vi "GPI-Join Sequences.vi"() -> ()   [LabVIEW 2015]
doc: "Combines two Glimpse video sequences into a single sequence that has the frames in chronological order based on time stamps."
uses:
  Header2 file data.ctl
  GLIMPSE Globals.vi
panel:
  in  "Number of acquisition files":i32=10
  out "Input Sequences Progress (%)":dbl[](array[slide]) scale=0.0..100.0
  out "Output frame number":i32(slide) scale=0.0..68.0
  in  "Radio Buttons":enum32{"New button", "Over-write button"}(radio)
  in  "Save into new directory:":path=path "d:/1.glimpse"
  in  "Over-write exisitng:":path=path "d:/1.glimpse"
  in  "Sequences to Join":path[](array[path])
  in  "Exit":bool
  in  "Go!":bool
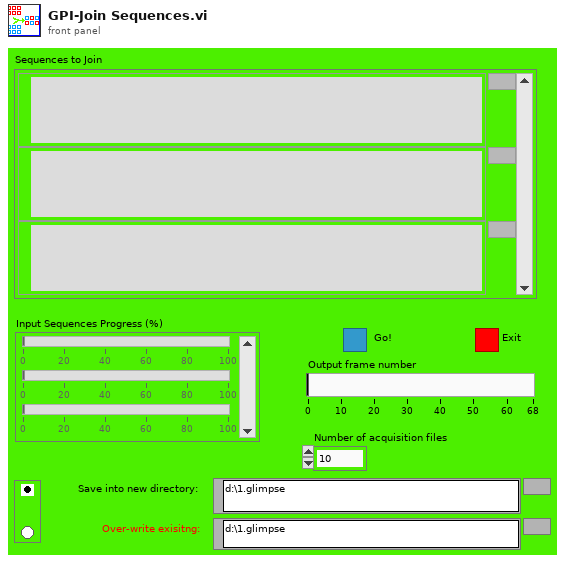
[diagram p1: front panel]
types:
  T1 = typedef "Header2 file data.ctl" = cluster{"Camera":string, "Microscope":string, "Microscope software version":string, "Laser names":string[], "Filter names":string[], "Lasers array":u16[][], "Filter array":u16[], "Flow rate array":dbl[], "Temperature array":dbl[], "Field array":u16[], "Is header2 info present?":bool, "Description Info":string, "Stage xyz array":dbl[][]}
  T2 = typedef "Header file data.ctl" = cluster{"Frames Acquired":u32, "Region width":i32, "Region height":i32, "Element 0 of TTB":u32, "time of 1st frame, \nsec since 1/1/04":dbl, "TTB Array (ms)":u32[], "Offsets Array":T3, "Pixel depth":u32}
  T3 = typedef "Offset table.ctl" = cluster{"offset":T4, "file number":T5}[]
  T4 = typedef "Offset.ctl" = i32
  T5 = typedef "file number.ctl" = u8
  T6 = typedef "IMAQ Image.ctl" = refnum<image>
  T7 = typedef "Sequence files handle.ctt" = cluster{"Sequence files directory path":path, "Sequence files refnum array":refnum<file>[]}
  T8 = typedef "Image Type" = u32
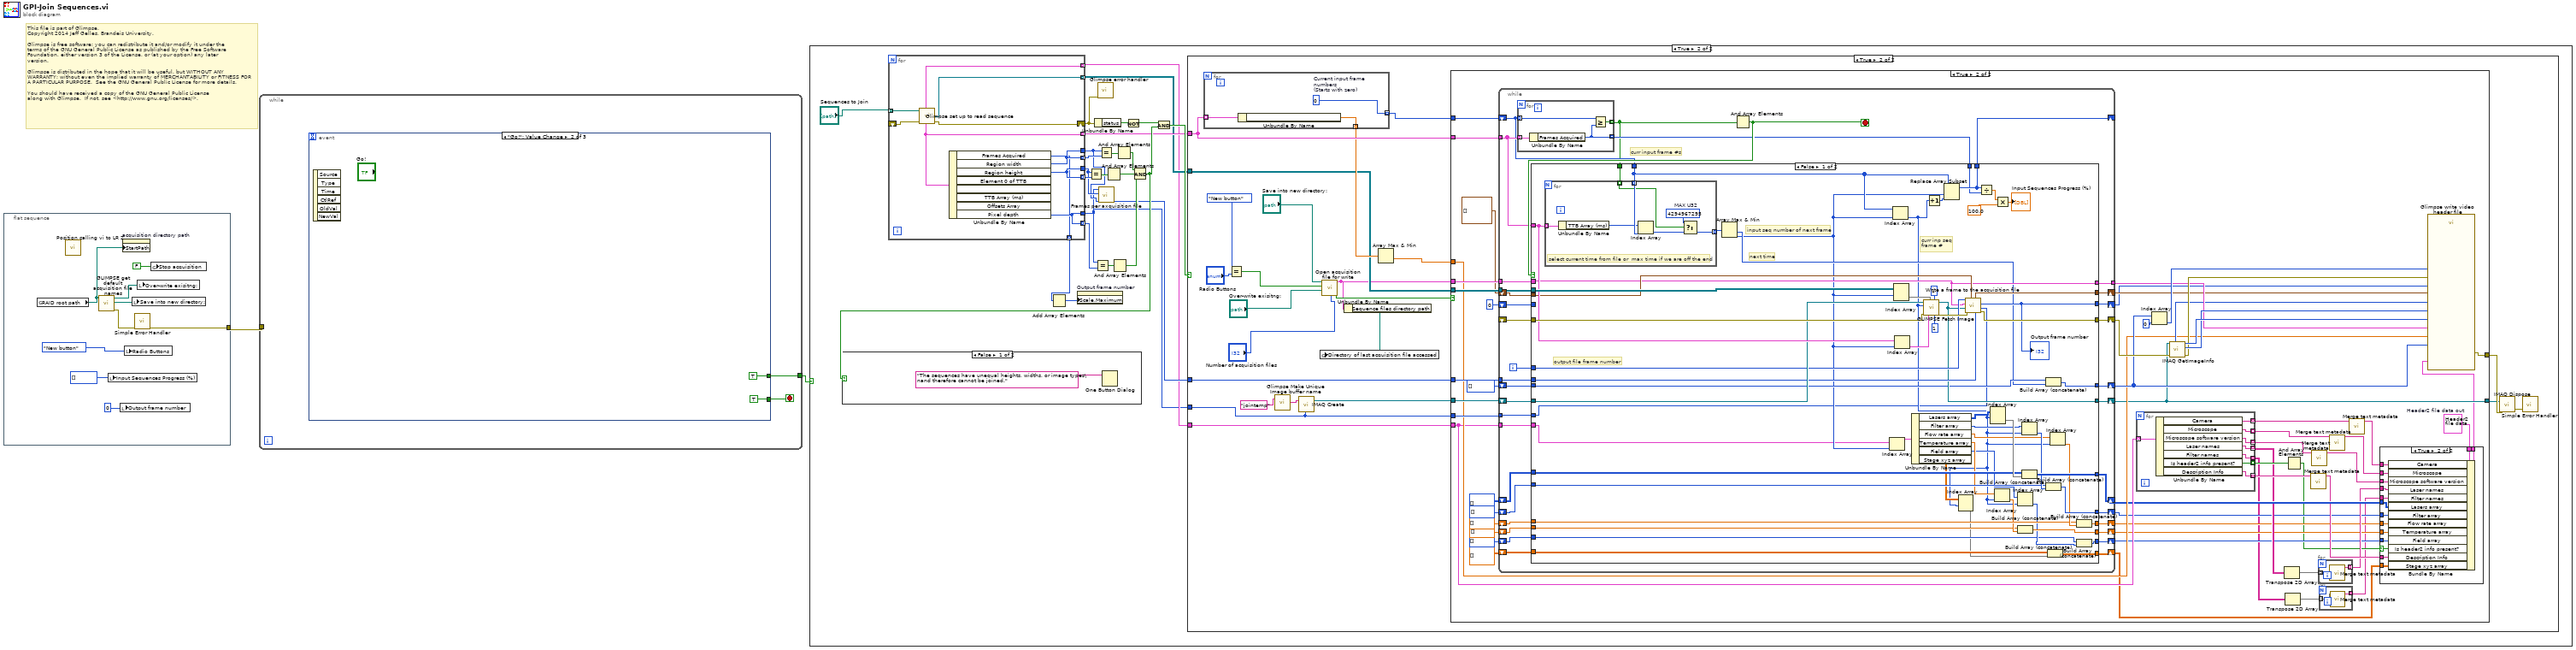
[diagram p0: block diagram]
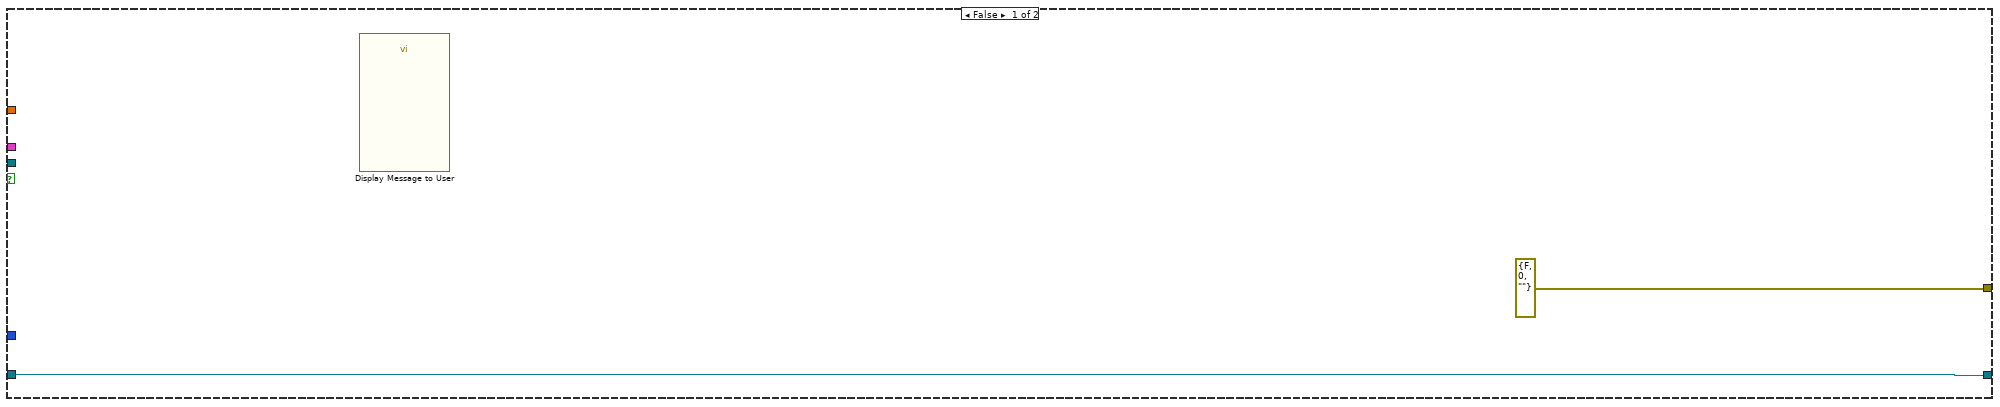
[diagram p4: hidden frame]
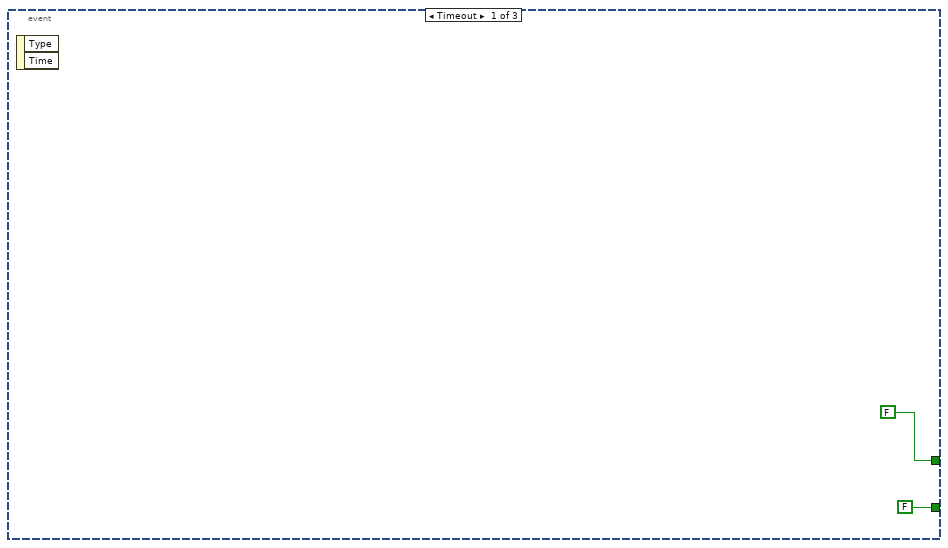
[diagram p8: hidden frame]
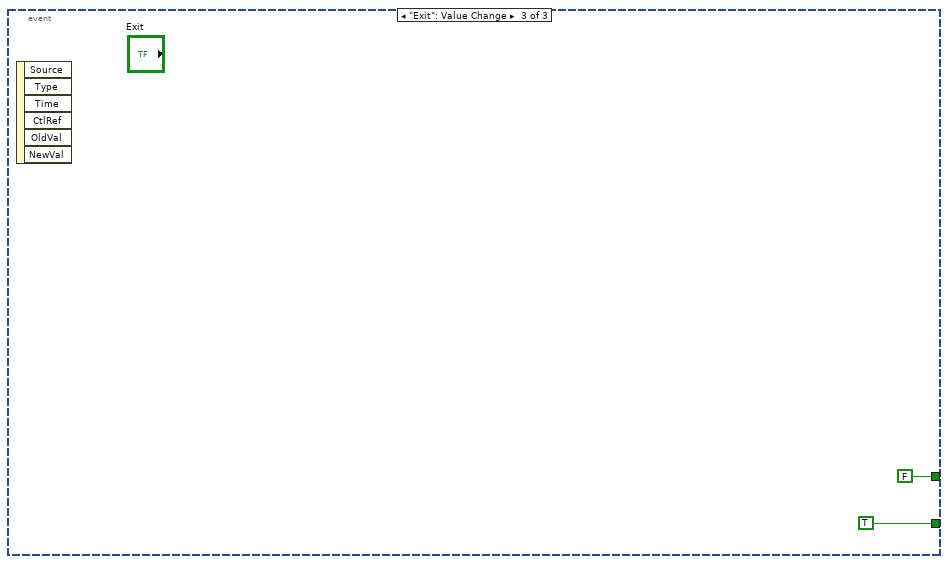
[diagram p9: hidden frame]
diagram:
  # "This file is part of Glimpse. \nCopyright 2014 Jeff Gelles, Brandeis University.    \n\nGlimpse is free software: you can redistribute it and/or modify it under the \nterms of the GNU General Public License as published by the Free Software \nFoundation, either version 3 of the License, or (at your option) any later \nversion.\n\nGlimpse is distributed in the hope that it will be useful, but WITHOUT ANY \nWARRANTY; without even the implied warranty of MERCHANTABILITY or FITNESS FOR \nA PARTICULAR PURPOSE.  See the GNU General Public License for more details.\n\nYou should have received a copy of the GNU General Public License\nalong with Glimpse.  If not, see <http://www.gnu.org/licenses/>."
  n1 = flat-sequence {
    tunnel: [w6] -> w1
    frame #0 {
      n2 = global read "GLIMPSE Globals.vi" "RAID root path"() -> (w3:path)
      n3 = call "Position calling vi to LR 2.vi"() -> ()  [unwired: 2 in, 4 out]
      n4 = call "GLIMPSE get default acquisition file names.vi"("RAID root path"=w3) -> ("error out"=w9:errorcluster, "next directory path"=w10:path, "last directory path"=w11:path)  [unwired: 1 in, 5 out]
      n5 = local write "Input Sequences Progress (%)"(u64[] [] ("Input Sequences Progress (%)")) -> ()
      n6 = local write "Output frame number"(0 ("Output frame number")) -> ()
      n7 = property on="acquisition directory path" class="Path"("StartPath"=w3) -> ()  [unwired: 2 in, 2 out]
      n8 = local write "Radio Buttons"(enum32{"New button", "Over-write button"}."New button" ("Radio Buttons")) -> ()
      n9 = local write "Save into new directory:"(w10) -> ()
      n10 = call <vilib>:"Simple Error Handler.vi"("error in (no error)"=w9) -> ("error out"=w6:errorcluster)  [unwired: 1 in, 7 out]
      n11 = local write "Over-write exisitng:"(w11) -> ()
      n12 = global write "GLIMPSE Globals.vi" "Stop acquisition"(FALSE ("Stop acquisition")) -> ()
    }
  }
  n13 = while {
    tunnel: [w12] -> w2
    tunnel: w1 -> [_]
    stop <- w13 stop-if-true
    n14 = event shown="[1] \"Go!\": Value Change" {
      selector: _ -> [_ _ _]
      dyn-events: _ -> [_ _ _]
      timeout: _ -> [_ _ _]
      tunnel: [FALSE TRUE TRUE] -> w13
      tunnel: [FALSE ("Boolean") TRUE FALSE] -> w12
      event Timeout {
        n15 = event-data() -> ()  [unwired: 3 out]
      }
      event "Go!": Value Change {
        n16 = event-data() -> ()  [unwired: 7 out]
      }
      event "Exit": Value Change {
        n17 = event-data() -> ()  [unwired: 7 out]
      }
    }
  }
  n18 = case shown="True" w2 {
    frame False {
    }
    frame True {
      n19 = for {
        tunnel: "Sequences to Join" -> [w282] mode=indexing
        shift-right: [w280] -> w33
        shift-left: _ -> [w281]
        tunnel: [w279] -> w29 mode=indexing
        tunnel: [w278] -> w26
        tunnel: [w277] -> w27
        tunnel: [w276] -> w37 mode=indexing
        tunnel: [w278] -> w42 mode=indexing
        tunnel: [w277] -> w39 mode=indexing
        tunnel: [w276] -> w20
        tunnel: [w275] -> w28 mode=indexing
        tunnel: [w274] -> w23 mode=indexing
        tunnel: [w273] -> w21 mode=indexing
        n20 = call "Glimpse set up to read sequence.vi"("acquisition directory path"=w282, "error in"=w281) -> ("Header2 file data out"=w273:T1, "Header file data out"=w279:T2, "Acquisition refnum array"=w275:refnum<file>[], "error out"=w280:errorcluster)  [unwired: 2 out]
        n21 = Unbundle By Name(w279) -> ("Frames Acquired"=w274:u32, "Region width"=w278:i32, "Region height"=w277:i32, "Pixel depth"=w276:u32)  [unwired: 4 out]
      }
      n22 = Add Array Elements(numeric array=w23) -> (sum=w24:u32)
      n23 = property on="Output frame number" class="Slide (strict)"("Scale.Maximum"=w24) -> ()  [unwired: 2 in, 2 out]
      n24 = Equal?(x=w27, y=w39) -> (x = y?=w40:bool[])
      n25 = Unbundle By Name(w33) -> ("status"=w32:bool)
      n26 = Equal?(x=w20, y=w37) -> (x = y?=w38:bool[])
      n27 = call "Glimpse error handler.vi"("error in"=w33) -> ()  [unwired: 1 in, 6 out]
      n28 = call "Frames per axquisition file.vi"("Output frame width"=w26, "Output frame height"=w27, "Pixel depth"=w20) -> ("Frames per acquisition file"=w25:i32)  [unwired: 3 in, 1 out]
      n29 = Equal?(x=w26, y=w42) -> (x = y?=w41:bool[])
      n30 = And Array Elements(Boolean array=w40) -> (logical AND=w35:bool)
      n31 = And Array Elements(Boolean array=w38) -> (logical AND=w36:bool)
      n32 = And Array Elements(Boolean array=w41) -> (logical AND=w34:bool)
      n33 = Not(x=w32) -> (.not. x?=w22:bool)
      n34 = Compound Arithmetic op=AND(w34, w35, w36) -> (w31:bool)
      n35 = case shown="False" w31 {
        frame False {
          n36 = One Button Dialog(message="The sequences have unequal heights, widths, or image types\nand therefore cannot be joined.") -> ()  [unwired: 2 out]
        }
        frame True {
        }
      }
      n37 = And(x=w22, y=w31) -> (x .and. y?=w30:bool)
      n38 = case shown="True" w30 {
        tunnel: w29 -> [_ w59]
        tunnel: w28 -> [_ w57]
        tunnel: w20 -> [_ w53]
        tunnel: w25 -> [_ w52]
        tunnel: w21 -> [_ w45]
        frame False {
        }
        frame True {
          n39 = for {
            tunnel: [w271] -> w66 mode=indexing
            tunnel: w59 -> [w270] mode=indexing
            tunnel: [w269] -> w58 mode=indexing
            w271 = u64 0  # Current input frame  numbers (Starts with zero)
            n40 = Unbundle By Name(w270) -> ("time of 1st frame, \nsec since 1/1/04"=w269:dbl)
          }
          n41 = Equal?(x=enum32{"New button", "Over-write button"}."New button", y="Radio Buttons") -> (x = y?=w61:bool)
          n42 = call "Glimpse Make Unique Image buffer name.vi"("Buffer  base name"="jointemp" ("Image Name")) -> ("Image Name"=w56:string)  [unwired: 1 out]
          n43 = call "IMAQ Create"("Image Name"=w56, "Image Type"=w53) -> ("New Image"=w54:T6)  [unwired: 2 in, 2 out]
          n44 = call "Open acquisition file for write.vi"("Number of acquisition files"="Number of acquisition files", "Existing directory to over-write"="Over-write exisitng:", "Use new?"=w61, "New directory to create"="Save into new directory:") -> ("OK?"=w60:bool, "Sequence files handle"=w47:T7)  [unwired: 5 out]
          n45 = Unbundle By Name(w47) -> ("Sequence files directory path"=w46:path)
          n46 = global write "GLIMPSE Globals.vi" "Directory of last acquisition file accessed"(w46) -> ()
          n47 = Array Max & Min(array=w58) -> (min value=w51:dbl)  [unwired: 3 out]
          n48 = case shown="True" w60 {
            tunnel: w66 -> [_ w123]
            tunnel: w59 -> [_ w122]
            tunnel: w57 -> [_ w121]
            tunnel: w54 -> [w68 w120]
            tunnel: w47 -> [_ w119]
            tunnel: w53 -> [_ w118]
            tunnel: w52 -> [_ w116]
            tunnel: w51 -> [_ w103]
            tunnel: [errorcluster {"status"=FALSE, "code"=0, "source"=""} ("error out") w102] -> w50
            tunnel: [w68 w101] -> w49
            tunnel: w45 -> [_ w99]
            frame False {
              n49 = call "Display Message to User"() -> ()  [unwired: 3 in, 9 out]
            }
            frame True {
              w97 = T1 {"Camera"="", "Microscope"="", "Microscope software version"="", "Laser names"=[], "Filter names"=[], "Lasers array"=[], "Filter array"=[], "Flow rate array"=[], "Temperature array"=[], "Field array"=[], "Is header2 info present?"=FALSE, "Description Info"="", "Stage xyz array"=[]}  # Header2 file data out
              n50 = while {
                tunnel: w122 -> [w185]
                shift-right: [w173] -> _
                shift-left: w123 -> [w184]
                tunnel: w121 -> [w183]
                shift-right: [w181] -> w111
                shift-left: _ -> [w182]
                shift-right: [w172] -> w101
                shift-left: w120 -> [w180]
                tunnel: w119 -> [w179]
                tunnel: w118 -> [w177]
                shift-right: [w176] -> w104
                shift-left: cluster{"offset":i32, "file number":u8}[] [] ("Offset table out") -> [w175]
                tunnel: w116 -> [w174]
                shift-right: [w171] -> w107
                shift-left: u32[] [] -> [w170]
                shift-right: [w169] -> w100
                shift-left: u32 0 ("Last frame number written out") -> [w168]
                tunnel: [w167] -> w106
                tunnel: w99 -> [w165]
                shift-right: [w164] -> w90
                shift-left: u16[][] [] -> [w163]
                shift-right: [w162] -> w83
                shift-left: u16[] [] -> [w161]
                shift-right: [w160] -> w82
                shift-left: dbl[] [] -> [w159]
                shift-right: [w158] -> w81
                shift-left: dbl[] [] -> [w157]
                shift-right: [w156] -> w80
                shift-left: u16[] [] -> [w155]
                shift-right: [w153] -> w75
                shift-left: dbl[][] [] -> [w154]
                i -> [w178]
                stop <- w186 stop-if-true
                # "curr input frame #s"
                n51 = for {
                  tunnel: w184 -> [w265] mode=indexing
                  tunnel: w185 -> [w268] mode=indexing
                  tunnel: [w267] -> w152 mode=indexing
                  tunnel: [w266] -> w166 mode=indexing
                  n52 = Unbundle By Name(w268) -> ("Frames Acquired"=w266:u32)
                  n53 = Greater Or Equal?(x=w265, y=w266) -> (x >= y?=w267:bool)
                }
                n54 = And Array Elements(Boolean array=w152) -> (logical AND=w186:bool)
                n55 = case shown="False" w186 {
                  tunnel: w185 -> [w238 _]
                  tunnel: w184 -> [w229 w258]
                  tunnel: w183 -> [w243 _]
                  tunnel: w182 -> [w241 w262]
                  tunnel: [w234 w262] -> w181
                  tunnel: w180 -> [w236 w260]
                  tunnel: w179 -> [w224 w259]
                  tunnel: w178 -> [w233 _]
                  tunnel: w177 -> [w188 _]
                  tunnel: [w232 w264] -> w176
                  tunnel: w175 -> [w231 w264]
                  tunnel: w174 -> [w230 _]
                  tunnel: [w223 w258] -> w173
                  tunnel: [w227 w260] -> w172
                  tunnel: [w226 w261] -> w171
                  tunnel: w170 -> [w225 w261]
                  tunnel: [w218 w263] -> w169
                  tunnel: w168 -> [_ w263]
                  tunnel: [w224 w259] -> w167
                  tunnel: w166 -> [w222 _]
                  tunnel: w165 -> [w214 _]
                  tunnel: [w211 w257] -> w164
                  tunnel: w163 -> [w210 w257]
                  tunnel: [w207 w256] -> w162
                  tunnel: w161 -> [w206 w256]
                  tunnel: [w197 w255] -> w160
                  tunnel: w159 -> [w203 w255]
                  tunnel: [w201 w254] -> w158
                  tunnel: w157 -> [w199 w254]
                  tunnel: [w196 w253] -> w156
                  tunnel: w155 -> [w194 w253]
                  tunnel: w154 -> [w193 w252]
                  tunnel: [w189 w252] -> w153
                  tunnel: w152 -> [w187 _]
                  frame False {
                    # "output file frame number"
                    # "curr inp seq\nframe #"
                    # "input seq number of next frame"
                    # "next time"
                    n56 = for {
                      tunnel: w238 -> [w251] mode=indexing
                      tunnel: w229 -> [w250] mode=indexing
                      tunnel: [w247] -> w244 mode=indexing
                      tunnel: w187 -> [w246] mode=indexing
                      w245 = u32 4294967295  # MAX U32
                      # "select current time from file or  max time if we are off the end"
                      n57 = Unbundle By Name(w251) -> ("TTB Array (ms)"=w249:u32[])
                      n58 = Index Array(array=w249, index=w250) -> (element=w248:u32)
                      n59 = Select(t=w245, s=w246, f=w248) -> (s? t:f=w247:u32)
                    }
                    n60 = Array Max & Min(array=w244) -> (min value=w217:u32, min index (indices)=w216:i32)  [unwired: 2 out]
                    n61 = Index Array(array=w214, index=w216) -> (element=w215:T1)
                    n62 = Index Array(array=w229, index=w216) -> (element=w191:u64)
                    n63 = Index Array(array=w243, index (row)=w216) -> (element=w242:refnum<file>[])  [unwired: 1 in]
                    n64 = Index Array(array=w238, index=w216) -> (element=w237:T2)
                    n65 = Unbundle By Name(w215) -> ("Lasers array"=w213:u16[][], "Filter array"=w209:u16[], "Flow rate array"=w205:dbl[], "Temperature array"=w202:dbl[], "Field array"=w198:u16[], "Stage xyz array"=w192:dbl[][])
                    n66 = call "GLIMPSE Fetch Image.vi"("Display FOV number"=i16 1, "Total FOVs"=i16 1, "Header file data"=w237, "Acqisition files refnums"=w242, "error in"=w241, "Logical Frame Number\n(starting with zero)"=w191, "Image In"=w236) -> ("error out"=w235:errorcluster, "Image Out"=w227:T6)  [unwired: 2 in, 1 out]
                    n67 = Increment(x=w191) -> (x+1=w228:u64)
                    n68 = Replace Array Subset(array=w229, new element=w228, index=w216) -> (w223:u64[])
                    n69 = Index Array(array=w192, index (row)=w191) -> (element=w190:dbl[])  [unwired: 1 in]
                    n70 = call "Write a frame to the acquisition file.vi"("Pixel depth"=w188, "Frames per acquisition file"=w230, "Offset table in"=w231, "error in"=w235, "Image In"=w227, "Sequence files handle"=w224, "Last frame number written in"=w233) -> ("error out"=w234:errorcluster, "Last frame number written out"=w218:u32, "Offset table out"=w232:T3)  [unwired: 2 out]
                    "Output frame number" <- w218
                    n71 = Divide(x=w223, y=w222) -> (x/y=w221:dbl[])
                    n72 = Index Array(array=w213, index (row)=w191) -> (element=w212:u16[])  [unwired: 1 in]
                    n73 = Index Array(array=w202, index=w191) -> (element=w200:dbl)
                    n74 = Multiply(x=w221, y=100.0) -> (x*y=→"Input Sequences Progress (%)":dbl[])
                    n75 = Index Array(array=w198, index=w191) -> (element=w195:u16)
                    n76 = Build Array (concatenate)(w199, w200) -> (w201:dbl[])
                    n77 = Index Array(array=w209, index=w191) -> (element=w208:u16)
                    n78 = Build Array (concatenate)(w210, w212) -> (w211:u16[][])
                    n79 = Build Array (concatenate)(w225, w217) -> (w226:u32[])
                    n80 = Build Array (concatenate)(w206, w208) -> (w207:u16[])
                    n81 = Build Array (concatenate)(w193, w190) -> (w189:dbl[][])
                    n82 = Index Array(array=w205, index=w191) -> (element=w204:dbl)
                    n83 = Build Array (concatenate)(w203, w204) -> (w197:dbl[])
                    n84 = Build Array (concatenate)(w194, w195) -> (w196:u16[])
                  }
                  frame True {
                  }
                }
              }
              n85 = for {
                tunnel: w99 -> [w151] mode=indexing
                tunnel: [w150] -> w98 mode=indexing
                tunnel: [w149] -> w94 mode=indexing
                tunnel: [w148] -> w91 mode=indexing
                tunnel: [w147] -> w85 mode=indexing
                tunnel: [w146] -> w88 mode=indexing
                tunnel: [w145] -> w70 mode=indexing
                tunnel: [w144] -> w86 mode=indexing
                n86 = Unbundle By Name(w151) -> ("Camera"=w150:string, "Microscope"=w149:string, "Microscope software version"=w148:string, "Laser names"=w147:string[], "Filter names"=w145:string[], "Is header2 info present?"=w144:bool, "Description Info"=w146:string)
              }
              n87 = Index Array(array=w107, index=0) -> (element=w108:u32)
              n88 = call "IMAQ GetImageInfo"("error in (no error)"=w111, "Image"=w101) -> ("error out"=w110:errorcluster, "Y Resolution"=w112:i32, "X Resolution"=w113:i32, "Image Type"=w105:T8)  [unwired: 6 out]
              n89 = Transpose 2D Array(2D array=w85) -> (transposed array=w72:string[][])
              n90 = Transpose 2D Array(2D array=w70) -> (transposed array=w71:string[][])
              n91 = And Array Elements(Boolean array=w86) -> (logical AND=w73:bool)
              n92 = call "Merge text metadata.vi"("Input metadata text array"=w88) -> ("Merged metadata text"=w87:string)  [unwired: 10 in]
              n93 = call "Merge text metadata.vi"("Input metadata text array"=w91) -> ("Merged metadata text"=w92:string)  [unwired: 10 in]
              n94 = for {
                tunnel: w72 -> [w143] mode=indexing
                tunnel: [w142] -> w84 mode=indexing
                n95 = call "Merge text metadata.vi"("Input metadata text array"=w143) -> ("Merged metadata text"=w142:string)  [unwired: 10 in]
              }
              n96 = for {
                tunnel: w71 -> [w125] mode=indexing
                tunnel: [w124] -> w69 mode=indexing
                n97 = call "Merge text metadata.vi"("Input metadata text array"=w125) -> ("Merged metadata text"=w124:string)  [unwired: 10 in]
              }
              n98 = call "Merge text metadata.vi"("Input metadata text array"=w94) -> ("Merged metadata text"=w93:string)  [unwired: 10 in]
              n99 = call "Merge text metadata.vi"("Input metadata text array"=w98) -> ("Merged metadata text"=w96:string)  [unwired: 10 in]
              n100 = case shown="True" w73 {
                selector: w73 -> [_ w127]
                tunnel: w97 -> [w126 w141]
                tunnel: w96 -> [_ w140]
                tunnel: [w126 w139] -> w95
                tunnel: w93 -> [_ w138]
                tunnel: w92 -> [_ w137]
                tunnel: w90 -> [_ w136]
                tunnel: w87 -> [_ w135]
                tunnel: w84 -> [_ w134]
                tunnel: w69 -> [_ w133]
                tunnel: w83 -> [_ w132]
                tunnel: w82 -> [_ w131]
                tunnel: w81 -> [_ w130]
                tunnel: w80 -> [_ w129]
                tunnel: w75 -> [_ w128]
                frame False {
                }
                frame True {
                  n101 = Bundle By Name(cluster=w141, "Camera"=w140, "Microscope"=w138, "Microscope software version"=w137, "Laser names"=w134, "Filter names"=w133, "Lasers array"=w136, "Filter array"=w132, "Flow rate array"=w131, "Temperature array"=w130, "Field array"=w129, "Is header2 info present?"=w127, "Description Info"=w135, "Stage xyz array"=w128) -> (w139:T1)
                }
              }
              n102 = call "Glimpse write video header file.vi"("Number of frames"=w100, "Sequence files handle"=w106, "Pixel depth\n(0=8 bit; 1= 16 bit)"=w105, "error in"=w110, "TTB Array"=w107, "Offsets Array"=w104, "Header2 file data"=w95, "Region width"=w113, "Region height"=w112, "Element 0 of TTB"=w108, "time of 1st frame, \nsec since 1/1/04"=w103) -> ("error out"=w102:errorcluster)  [unwired: 8 in]
            }
          }
          n103 = call "IMAQ Dispose"("Image"=w49, "error in (no error)"=w50) -> ("error out"=w48:errorcluster)  [unwired: 1 in, 3 out]
          n104 = call <vilib>:"Simple Error Handler.vi"("error in (no error)"=w48) -> ()  [unwired: 1 in, 8 out]
        }
      }
    }
  }
